vi "Write View Type.vi"(8 "error in (no error)":errorcluster, 10 "Event Actors.lvlib:View Actor.lvclass":refnum<class "View Actor.lvclass">, 11 "Example Controller Actor in":refnum<class "Example Controller Actor.lvclass">) -> (0 "error out":errorcluster, 3 "Example Controller Actor out":refnum<class "Example Controller Actor.lvclass">)   [LabVIEW 2017, in "Example Controller Actor.lvlib" / "Example Controller Actor.lvclass"]
uses:
  Example Controller Actor.lvclass
  View Actor/View Actor.lvclass
  Example Controller Actor.lvclass/Example Controller Actor.ctl
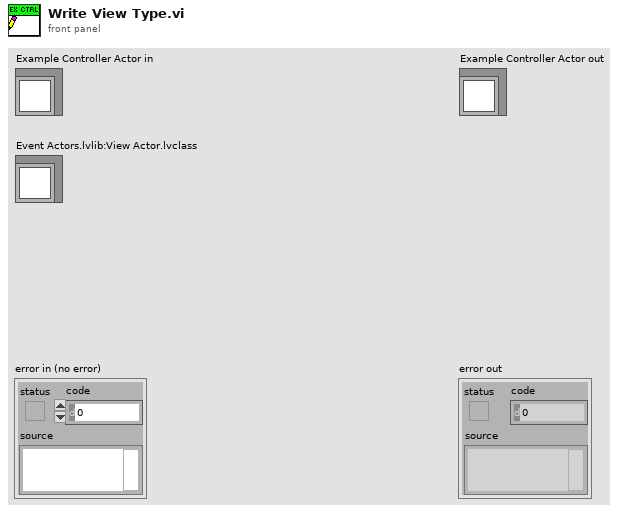
[diagram p1: front panel]
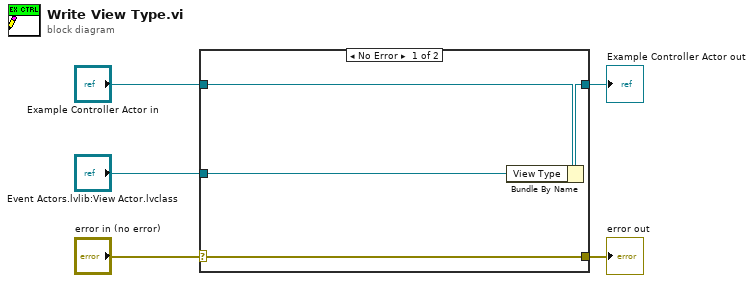
[diagram p0: block diagram]
diagram:
  n1 = case shown="No Error" "error in (no error)" {
    selector: "error in (no error)" -> [w9 w10]
    tunnel: [w9 w10] -> w4
    tunnel: [w7 w11] -> w2
    tunnel: "Example Controller Actor in" -> [w8 w11]
    tunnel: "Event Actors.lvlib:View Actor.lvclass" -> [w6 _]
    frame No Error {
      n2 = Bundle By Name(cluster=w8, "View Type"=w6) -> (w7:refnum<class "Example Controller Actor.lvclass">)
    }
    frame Error {
    }
  }
  "error out" <- w4
  "Example Controller Actor out" <- w2
